vi "Sets and Query the Calculate Function.vi"(5 "Enable to Query":bool=TRUE, 7 "Enable to Sets":bool=TRUE, 8 "error in":errorcluster, 10 "Calculate Function":u8(ring) items=["Off", "Minimum", "Maximum", "Hold", "Relative", "Compare", "dB", "dBm", "MX+B", "Inverse", "Reference"], 11 "VISA resource name":refnum<visa-resource-name>) -> (0 "error out":errorcluster, 2 "Return the Calculate Function":string, 3 "VISA resource name out":refnum<visa-resource-name>)   [LabVIEW 2011, in "DMM4.lvlib"]
uses:
  <instrlib>/DMM4/DMM4.lvlib
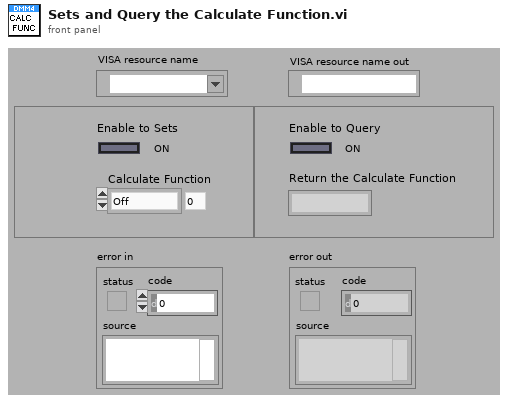
[diagram p1: front panel]
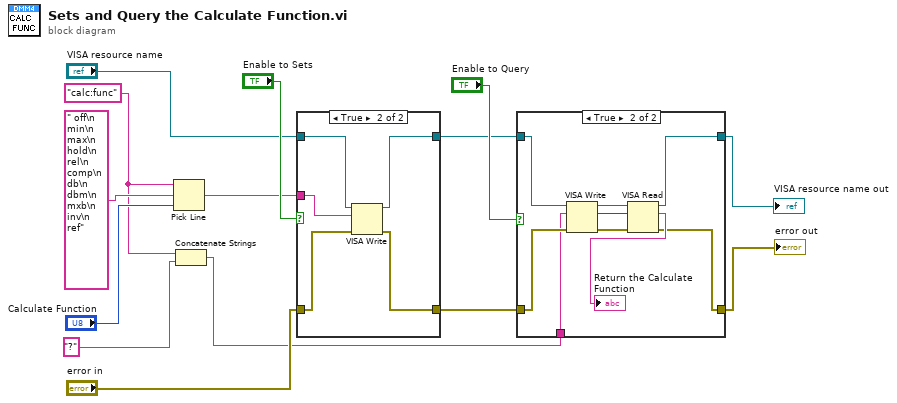
[diagram p0: block diagram]
diagram:
  w10 = "calc:func"
  n1 = Pick Line(string ("")=w10, multi-line string=" off\n min\n max\n hold\n rel\n comp\n db\n dbm\n mxb\n inv\n ref", line index="Calculate Function") -> (output string=w9:string)
  n2 = Concatenate Strings(w10, "?") -> (w3:string)
  n3 = case shown="True" "Enable to Sets" {
    tunnel: w9 -> [_ w21]
    tunnel: "VISA resource name" -> [w16 w20]
    tunnel: "error in" -> [w15 w19]
    tunnel: [w16 w18] -> w5
    tunnel: [w15 w17] -> w4
    frame False {
    }
    frame True {
      n4 = VISA Write(VISA resource name=w20, write buffer=w21, error in (no error)=w19) -> (VISA resource name out=w18:refnum<visa-resource-name>, error out=w17:errorcluster)  [unwired: 1 out]
    }
  }
  n5 = case shown="True" "Enable to Query" {
    tunnel: w5 -> [w23 w29]
    tunnel: w4 -> [w22 w28]
    tunnel: w3 -> [_ w27]
    tunnel: [w23 w25] -> w2
    tunnel: [w22 w24] -> w1
    frame False {
    }
    frame True {
      n6 = VISA Write(VISA resource name=w29, write buffer=w27, error in (no error)=w28) -> (VISA resource name out=w30:refnum<visa-resource-name>, return count=w31:u32, error out=w32:errorcluster)
      n7 = VISA Read(VISA resource name=w30, byte count=w31, error in (no error)=w32) -> (VISA resource name out=w25:refnum<visa-resource-name>, read buffer=→"Return the Calculate Function":string, error out=w24:errorcluster)  [unwired: 1 out]
    }
  }
  "VISA resource name out" <- w2
  "error out" <- w1
